vi "Compare Time.vi"(10 "TIEMPO DESEADO":dbl, 11 "Class 2.lvclass":refnum<class "Class 2.lvclass">) -> (1 "Numeric":dbl, 2 "validacion":bool, 3 "Class 2.lvclass 2":refnum<class "Class 2.lvclass">)   [LabVIEW 2019, in "Class 2.lvclass"]
uses:
  Class 2.lvclass
  Class 2.lvclass/Class 2.ctl
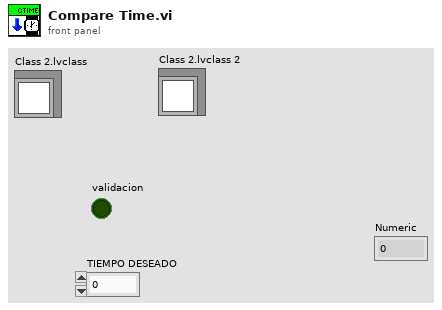
[diagram p1: front panel]
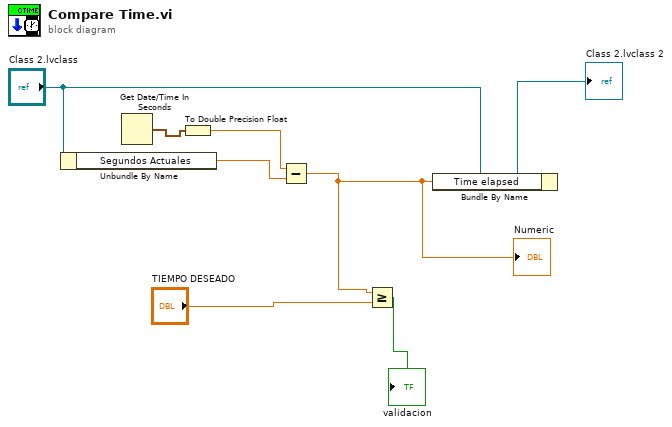
[diagram p0: block diagram]
diagram:
  n1 = Unbundle By Name("Class 2.lvclass") -> ("Segundos Actuales"=w3:dbl)
  n2 = Get Date/Time In Seconds() -> (seconds since 1Jan1904=w5:timestamp)
  n3 = To Double Precision Float(number=w5) -> (double precision float=w4:dbl)
  n4 = Subtract(x=w4, y=w3) -> (x-y=w2:dbl)
  "Numeric" <- w2
  n5 = Greater Or Equal?(x=w2, y="TIEMPO DESEADO") -> (x >= y?=→"validacion":bool)
  n6 = Bundle By Name(cluster="Class 2.lvclass", "Time elapsed"=w2) -> (→"Class 2.lvclass 2":refnum<class "Class 2.lvclass">)
